vi "Sort Serial Data.vi"(8 "error in":errorcluster, 11 "SerialData":refnum<class "Data.lvclass">[](array[class])) -> (0 "error out":errorcluster, 1 "acatDataOut":T2, 2 "TEC Data":T1)   [LabVIEW 2015]
doc: "This VI takes the array of serial data objects and extracts the data to the appropriate structures. This VI is necessary strictly for cleaning up the block diagram and is therefore set to inline for execution. During standard use the user will not be able to debug this VI so that the VI may be properly inlined by the compiler."
uses:
  Reusable/Data/Data.lvclass
  Devices/Alicat/Session Based/Data/Alicat Data.lvclass
  Devices/TE Cooler/Data/TECData.lvclass
  Devices/TE Cooler/Data/TECData.lvclass/TECData.ctl
  Devices/TE Cooler/Data/Data Access/Read Input 1.vi
  Devices/TE Cooler/Data/Data Access/Read Input 2.vi
  Devices/TE Cooler/Data/Data Access/Read Power.vi
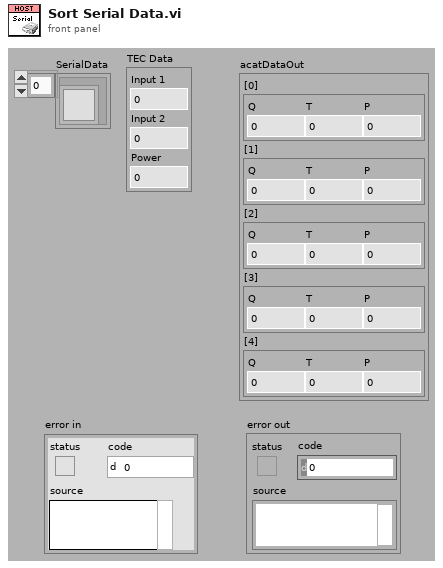
[diagram p1: front panel]
types:
  T1 = cluster{"Input 1":sgl, "Input 2":sgl, "Power":sgl}
  T2 = cluster{"[0]":cluster{"Q":sgl, "T":sgl, "P":sgl}, "[1]":cluster{"Q":sgl, "T":sgl, "P":sgl}, "[2]":cluster{"Q":sgl, "T":sgl, "P":sgl}, "[3]":cluster{"Q":sgl, "T":sgl, "P":sgl}, "[4]":cluster{"Q":sgl, "T":sgl, "P":sgl}}
  T3 = cluster{"Numeric":sgl, "Numeric":sgl, "Numeric":sgl}
  T4 = cluster{"[0]":cluster{"Numeric":sgl, "Numeric":sgl, "Numeric":sgl}, "[1]":cluster{"Numeric":sgl, "Numeric":sgl, "Numeric":sgl}, "[2]":cluster{"Numeric":sgl, "Numeric":sgl, "Numeric":sgl}, "[3]":cluster{"Numeric":sgl, "Numeric":sgl, "Numeric":sgl}, "[4]":cluster{"Numeric":sgl, "Numeric":sgl, "Numeric":sgl}}
  T5 = cluster{"Data Access:Input 1":sgl, "Data Access:Input 2":sgl, "Data Access:Power":sgl}
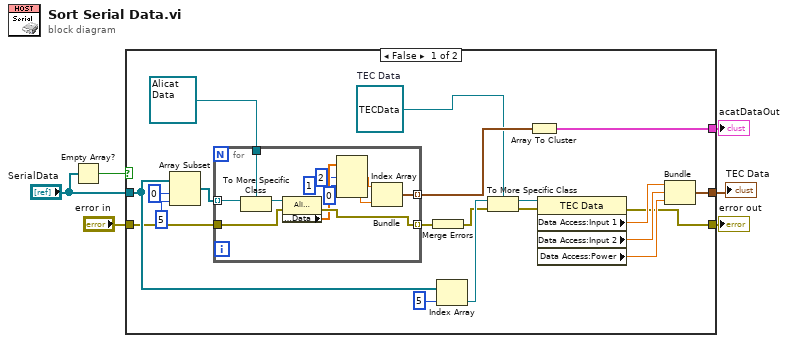
[diagram p0: block diagram]
diagram:
  n1 = Empty Array?(array="SerialData") -> (empty?=w4:bool)
  n2 = case shown="False" w4 {
    tunnel: "SerialData" -> [w22 _]
    tunnel: [w20 _] -> w6
    tunnel: [w9 w40] -> w2
    tunnel: "error in" -> [w18 w40]
    tunnel: [w10 _] -> w1
    frame False {
      w7 = refnum<class "TECData.lvclass"> refnum  # TEC Data
      n3 = Array Subset(array=w22, index=0, length=5) -> (w24:refnum<class "Data.lvclass">[])
      n4 = for {
        tunnel: w24 -> [w39] mode=indexing
        tunnel: refnum<class "Alicat Data.lvclass"> refnum ("Alicat Data") -> [w38]
        tunnel: [w37] -> w21 mode=indexing
        tunnel: [w34] -> w19 mode=indexing
        tunnel: w18 -> [w35]
        n5 = To More Specific Class(target class=w38, reference=w39) -> (specific class reference=w36:refnum<class "Alicat Data.lvclass">)  [unwired: 1 in, 1 out]
        n6 = property class="Alicat Data"(reference=w36, error in=w35) -> (error out=w34:errorcluster, "Accessors:Data"=w33:sgl[])  [unwired: 1 out]
        n7 = Index Array(array=w33, index #1=2 ("index"), index #2=1 ("index"), index #3=0 ("index")) -> (element #1=w29:sgl, element #2=w28:sgl, element #3=w27:sgl)
        n8 = Bundle("Numeric"=w29, "Numeric"=w28, "Numeric"=w27) -> (w37:T3)  [unwired: 1 in]
      }
      n9 = Merge Errors(w19) -> (w14:errorcluster)
      n10 = Index Array(array=w22, index=5) -> (element=w26:refnum<class "Data.lvclass">)
      n11 = To More Specific Class(target class=w7, reference=w26, error in=w14) -> (specific class reference=w16:refnum<class "TECData.lvclass">, error out=w15:errorcluster)
      n12 = Array To Cluster(array=w21) -> (cluster=w20:T4)
      n13 = property class="TEC Data"(reference=w16, error in=w15) -> (error out=w9:errorcluster, "Data Access:Input 1"=w13:sgl, "Data Access:Input 2"=w12:sgl, "Data Access:Power"=w11:sgl)  [unwired: 1 out]
      n14 = Bundle("Data Access:Input 1"=w13, "Data Access:Input 2"=w12, "Data Access:Power"=w11) -> (w10:T5)  [unwired: 1 in]
    }
    frame True {
    }
  }
  "acatDataOut" <- w6
  "error out" <- w2
  "TEC Data" <- w1
